vi "Thermal Chamber Controller_DQMH_Action Update Set Point-test_harness-Caraya.vi"(8 "error in (no error)":errorcluster) -> (0 "error out":errorcluster)   [LabVIEW 2018]
doc: "The harness VI is executed for every test case. InstaCoverage passes the test case ID before the execution of the test case in the <b>test case ID</b> input and reads the <b>result</b> output after the execution. If the result is TRUE and no error happens during the execution, then the test case is evaluated as PASSED. If the result is false and no error happens during the execution, then the test case is evaluated as FAILED. Otherwise the test case is evaluated as ERROR.\n\nThe result of the test suite will be PASSED (FAILED) if all (at least one) test cases are PASSED (FAILED). If at least one test case in the test suite has the ERROR result, then the test suite will have ERROR result.\n\n<b>Note: </b>Don't change the connector pane of this VI.\n\nSee the Help Document for more information. (<b>Help</b> > <b>IncQuery Labs</b> > <b>InstaCoverage</b> > <b>InstaCoverage Help...</b>)"
uses:
  <vilib>/addons/_JKI Toolkits/Caraya/classes/Assert/Assert True.vi
  Libraries/Thermal Chamber Controller_DQMH/Thermal Chamber Controller_DQMH.lvlib
  <vilib>/addons/_JKI Toolkits/Caraya/classes/Test/Test.lvclass
  <vilib>/addons/_JKI Toolkits/Caraya/classes/Assert/Assert.lvclass
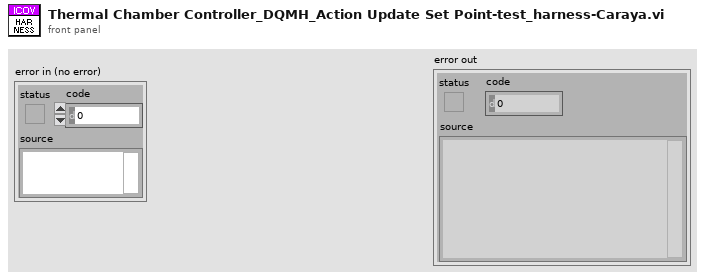
[diagram p1: front panel]
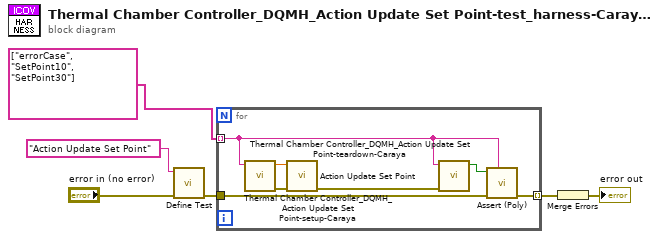
[diagram p0: block diagram]
diagram:
  n1 = call <vilib>:"Define Test.vi"("error in (no error)"="error in (no error)", "Label (VI Title)"="Action Update Set Point") -> ("error out"=w3:errorcluster)  [unwired: 9 in]
  n2 = for {
    tunnel: string[] ["errorCase", "SetPoint10", "SetPoint30"] -> [w7] mode=indexing
    tunnel: [w10] -> w4 mode=indexing
    tunnel: w3 -> [w9]
    n3 = call "Thermal Chamber Controller_DQMH_Action Update Set Point-setup-Caraya.vi"("test case ID"=w7) -> ("error in"=w12:errorcluster, "Temperature Set Point"=w13:dbl)  [unwired: 9 in]
    n4 = call "Action Update Set Point.vi"("error in (no error)"=w12, "Temperature Set Point"=w13) -> ("error out"=w11:errorcluster)  [unwired: 9 in]
    n5 = call "Thermal Chamber Controller_DQMH_Action Update Set Point-teardown-Caraya.vi"("error out"=w11, "test case ID"=w7) -> ("result"=w8:bool)  [unwired: 9 in]
    n6 = call-poly <vilib>:"Assert (Poly).vi"("Label"=w7, "error in (no error)"=w9, "True?"=w8) -> ("error out"=w10:errorcluster)  [unwired: 8 in]
  }
  n7 = Merge Errors(w4) -> (→"error out":errorcluster)
